vi "AD5781Standalone.vi"(9 "DacStateCmdByHost":T1, 10 "setDACRegister":u32=1048576 format="%024b") -> (1 "actDACRegister":u32=1572792 caption="actRegister" format="%024b", 2 "DacState":T1)   [LabVIEW 2014]
uses:
  Controls/DacState.ctl
  <vilib>/rvi/Emulation/niFpgaGetClockAttributes.vi
  <vilib>/rvi/Emulation/niFpgaSctlEmulationGetInTimedLoop.vi
  <vilib>/rvi/Emulation/niFpgaEmulationReportErrorSimple.vi
  Code/FPGA SPI_Globals.vi
  <vilib>/rvi/Emulation/niFpgaCriticalErrorInLSC.vi
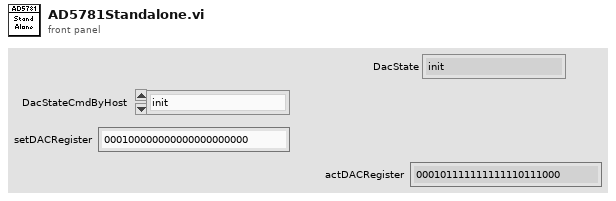
[diagram p1: front panel]
types:
  T1 = typedef "DacState.ctl" = enum16{"init", "idle", "setVolt", "error"}
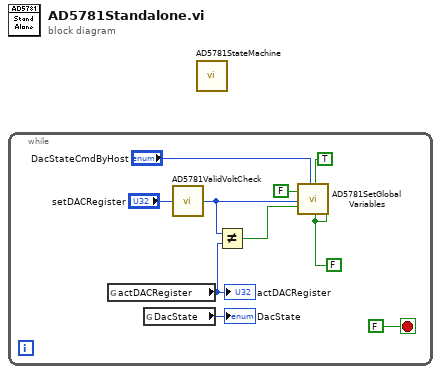
[diagram p0: block diagram]
diagram:
  n1 = while {
    stop <- FALSE stop-if-true
    w1 = FALSE ("write DacState")
    n2 = global read "FPGA SPI_Globals.vi" "actDACRegister"() -> (w6:u32)
    "actDACRegister" <- w6
    n3 = global read "FPGA SPI_Globals.vi" "DacState"() -> (→"DacState":T1)
    n4 = call "AD5781ValidVoltCheck.vi"("U32"="setDACRegister") -> ("coerced(x)"=w4:u32)  [unwired: 4 in]
    n5 = Not Equal?(x=w4, y=w6) -> (x != y?=w5:bool)
    n6 = call "AD5781SetGlobalVariables.vi"("write actDACRegister"=FALSE, "setDACRegister"=w4, "write setDACRegister"=w5, "DacStateCmdByHost"="DacStateCmdByHost", "write DacStateCmdByHost"=TRUE, "write DacState"=w1, "write dac0VRegister"=w1) -> ()  [unwired: 13 in]
  }
  n7 = call "AD5781StateMachine.vi"() -> ()  [unwired: 12 in]
